vi "Connection Handler Worker.vi"(9 "Additional Data":variant, 10 "connection ID":T1, 11 "TCP Server Refnum":refnum<class "JKI TCP Server.lvclass">) -> ()   [LabVIEW 2020, in "CSM-TCP-Router.lvlib"]
uses:
  CSM-TCP-Router.lvlib
  <vilib>/addons/_JKI.lib/_JKI_lib_TCP_Server.llb/TCP Server Connection Session ID Cluster.ctl
  <vilib>/addons/_JKI.lib/_JKI_lib_TCP_Server.llb/JKI TCP Server.lvclass
  typedef/tcp-msg type.ctl
  20ff867f-262a-4864-b042-c50abd455195.vi
  9f8653f6-ccbf-4dca-88e7-a4c531b7661f.vi
  bd168d05-2ccd-4f69-90c9-be1b4e621865.vi
  316abe05-dd11-44a4-98b3-32ea1594dc48.vi
  a7f8194b-54d4-448d-8a65-d0b66a8fd47c.vi
  8a9da1d4-9237-4126-a3a1-8a9d876b672d.vi
  eb58fbab-51b7-4bfd-aab6-475a21a34b28.vi
  66683ee4-8938-4a2b-95b9-1d8ed72716c9.vi
  <userlib>/_NEVSTOP/Communicable State Machine(CSM)/AdvanceAPI/CSM - Revert Arguments-Safe String.vi
  <userlib>/_NEVSTOP/Communicable State Machine(CSM)/_Support/Common/Trim Single line Text.vi
  <userlib>/_NEVSTOP/Communicable State Machine(CSM)/AdvanceAPI/CSM - Make String Arguments Safe.vi
  <userlib>/_NEVSTOP/Communicable State Machine(CSM)/AdvanceAPI/CSM - Compact Multiple States.vi
  <userlib>/_NEVSTOP/Communicable State Machine(CSM)/addons/API-String-Arugments-Support/_Support/Query Data as API String Arguments(variant).vi
  <userlib>/_NEVSTOP/Communicable State Machine(CSM)/AdvanceAPI/CSM - Keywords.vi
  <userlib>/_NEVSTOP/Communicable State Machine(CSM)/addons/API-String-Arugments-Support/_Support/Data To SingleElementsArray_with_itself_csm.vi
  <userlib>/_NEVSTOP/Communicable State Machine(CSM)/addons/API-String-Arugments-Support/_Support/Data To API String Arguments.vi
  <userlib>/_NEVSTOP/Communicable State Machine(CSM)/addons/API-String-Arugments-Support/_Support/Convert API String Arguments to Data(variant).vi
  <userlib>/_NEVSTOP/Communicable State Machine(CSM)/Communicable State Machine.lvlib
  <userlib>/_NEVSTOP/Communicable State Machine(CSM)/_csmHelper/API with lvcsm Support/CSM-Helper API with lvcsm Support.lvlib
panel:
  out "State History":string
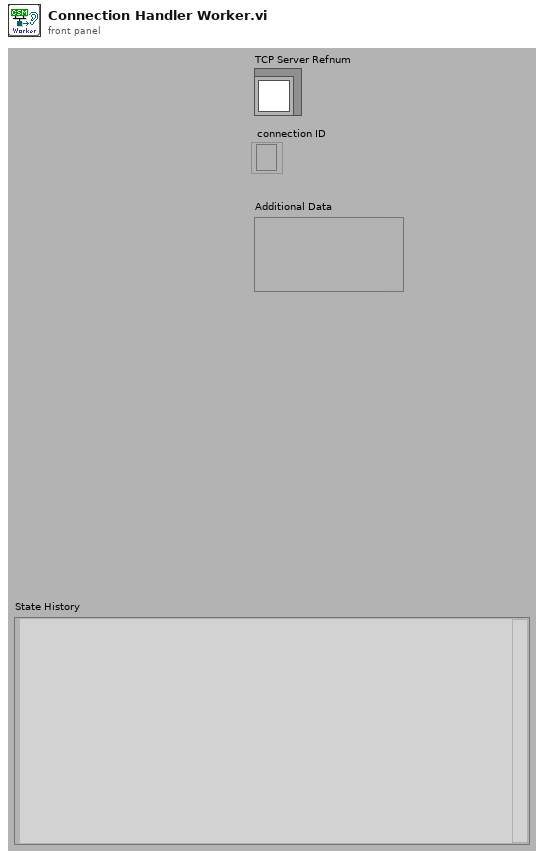
[diagram p1: front panel]
types:
  T1 = typedef "JKI TCP Server.lvclass/TCP Server Connection Session ID Cluster.ctl" = refnum<k5>
  T2 = typedef "CSM-TCP-Router.lvlib/tcp-msg type.ctl" = enum16{"info", "error", "cmd", "resp", "async-resp", "status", "interrupt"}
  T3 = enum32{"Invalid", "Standard", "Closed", "Hidden", "Minimized", "Maximized"}
  T4 = enum32{"invalid app kind", "Development System", "Run Time System", "Student Edition", "Embedded LabVIEW", "Evaluation", "Custom"}
  T5 = typedef "Communicable State Machine.lvlib/_CSM_Response Source Message.ctl" = cluster{"‘State":string, "’Arguments":string, "’Error":errorcluster}
  T6 = cluster{"Current VI Reference":refnum<vi>, "Close Panel on Exit?":bool}
  T7 = cluster{"Core":cluster{"Current VI Reference":refnum<vi>, "Close Panel on Exit?":bool}, "Your Boolean data":bool}
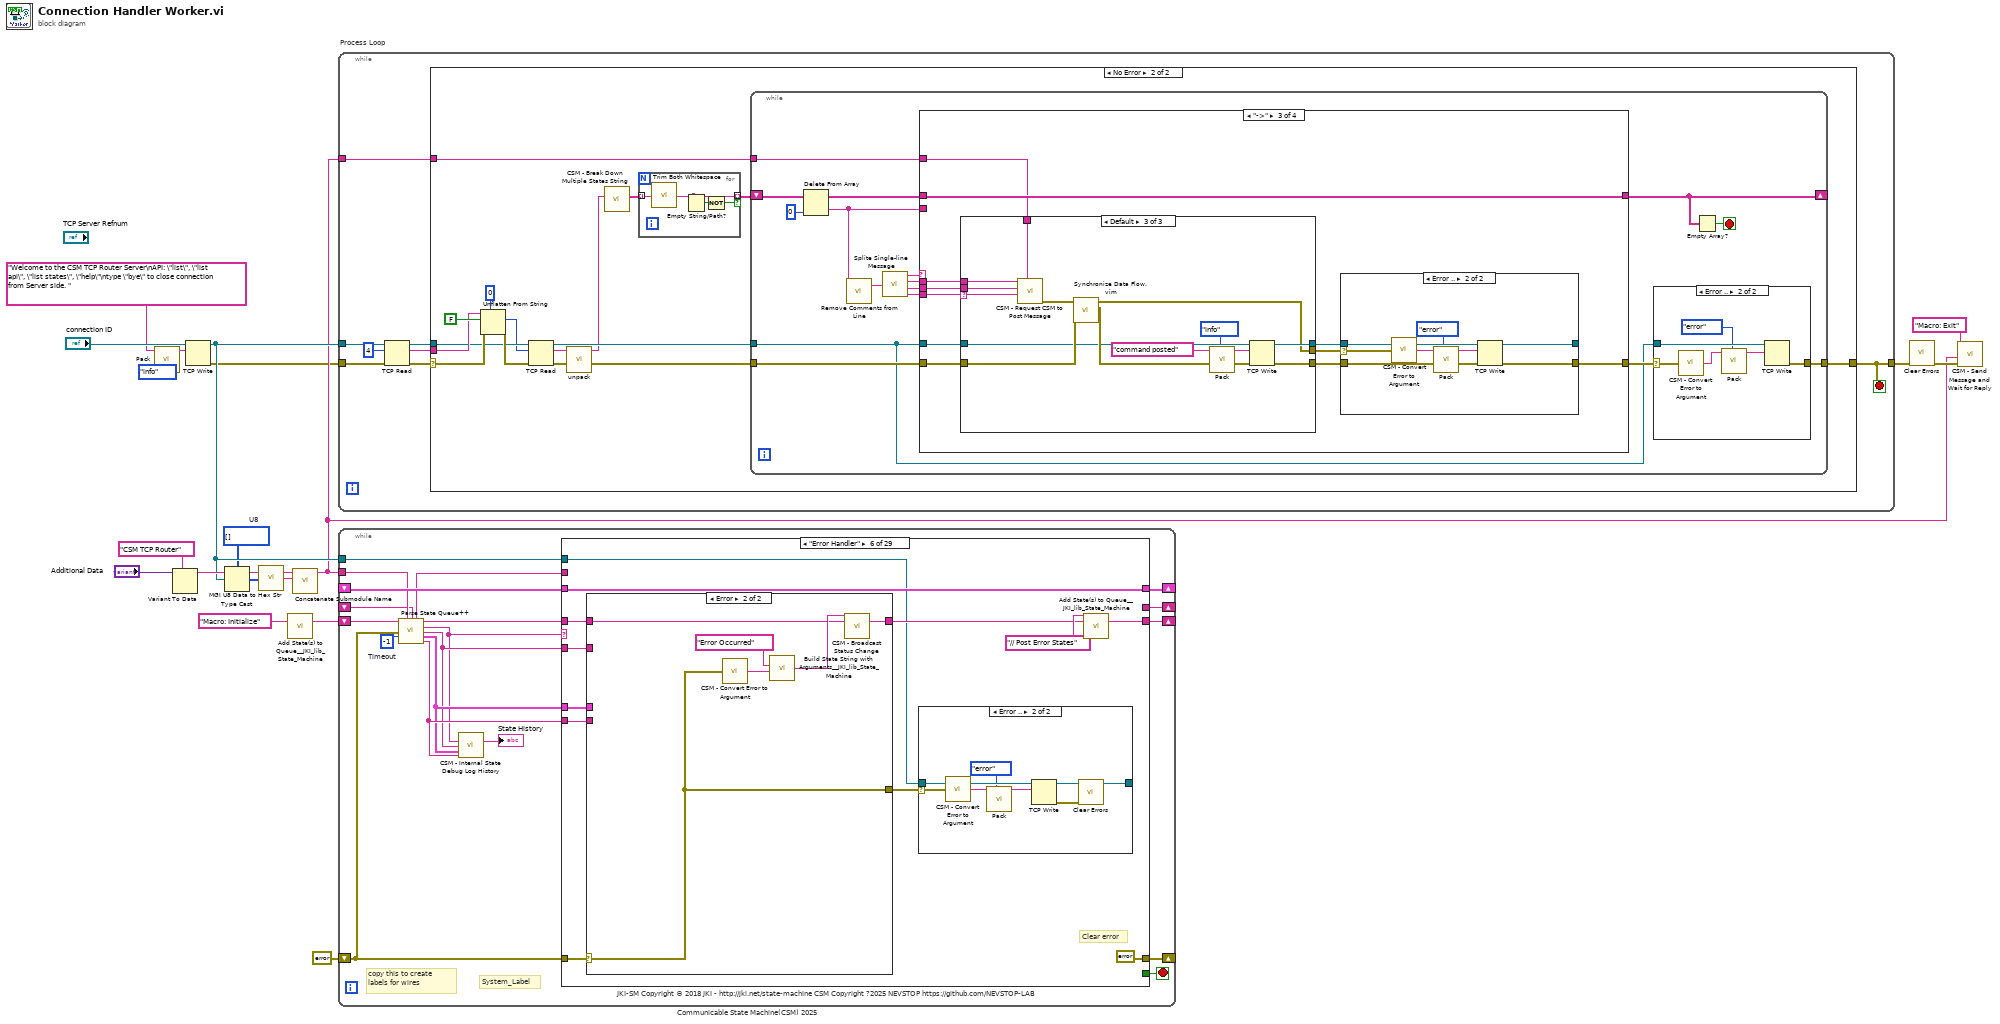
[diagram p0: block diagram]
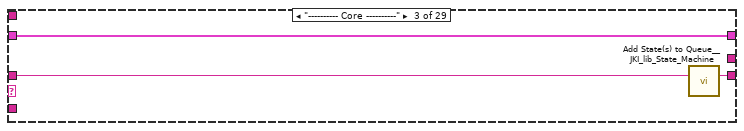
[diagram p4: hidden frame]
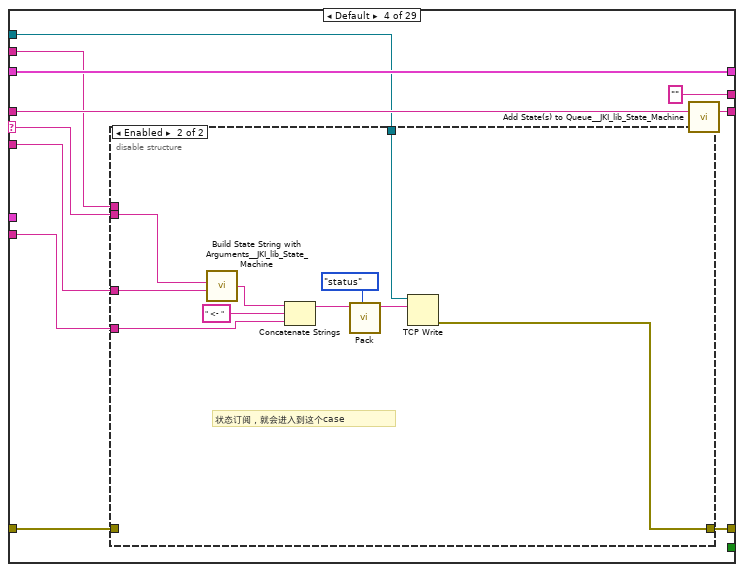
[diagram p5: hidden frame]
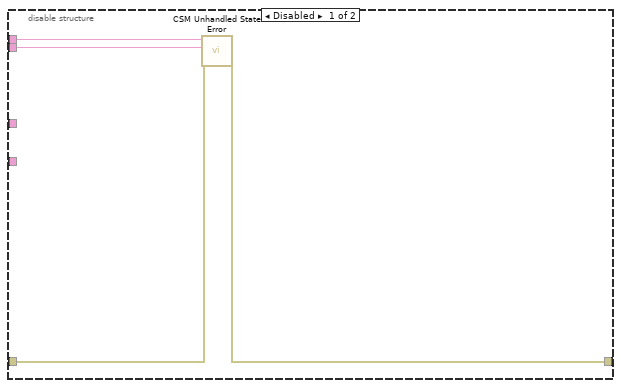
[diagram p6: hidden frame]
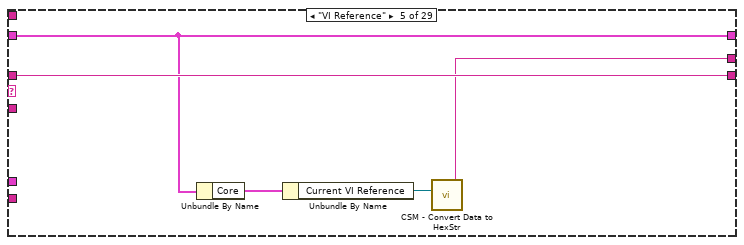
[diagram p7: hidden frame]
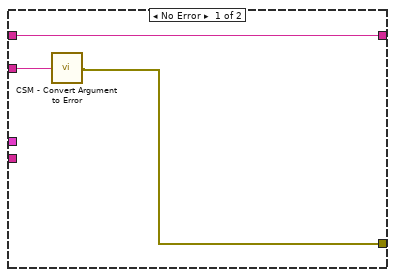
[diagram p9: hidden frame]
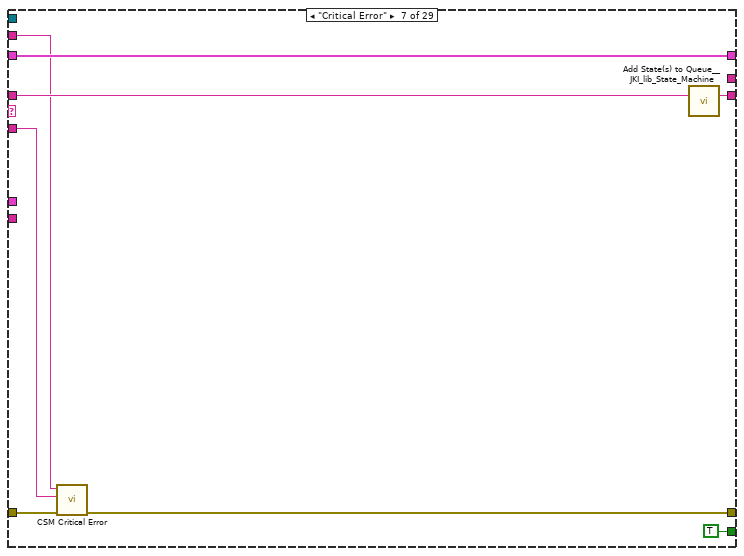
[diagram p10: hidden frame]
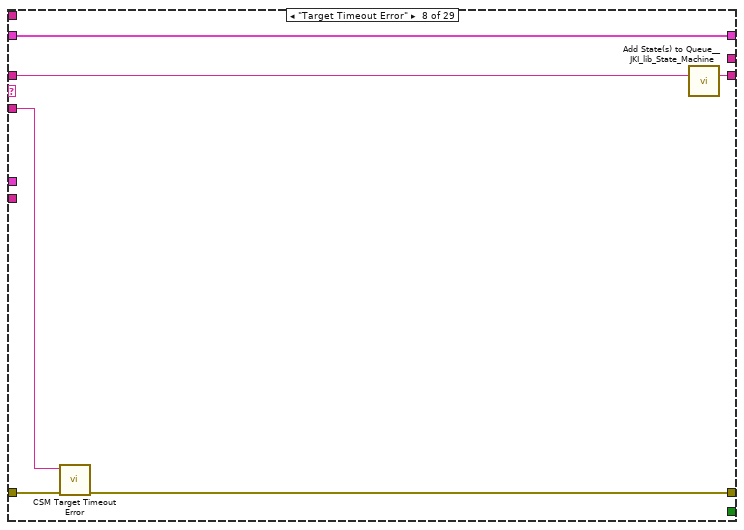
[diagram p11: hidden frame]
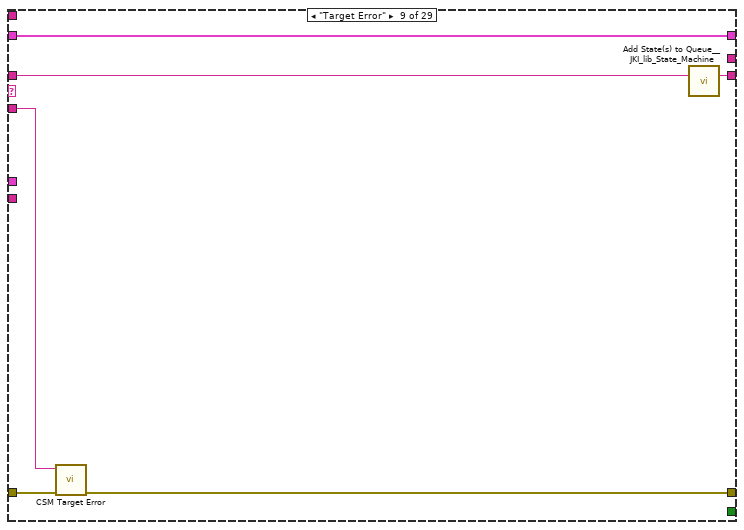
[diagram p12: hidden frame]
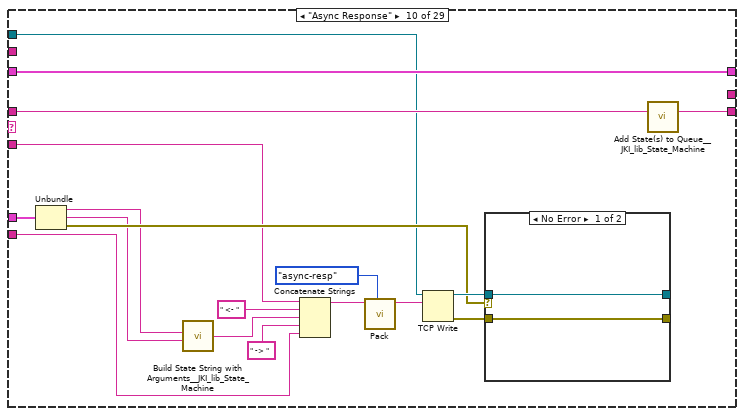
[diagram p13: hidden frame]
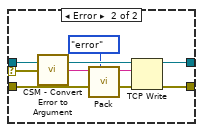
[diagram p14: hidden frame]
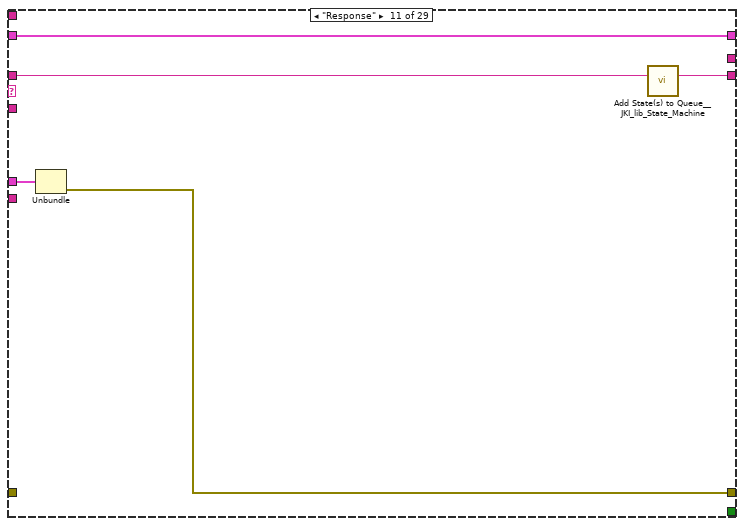
[diagram p15: hidden frame]
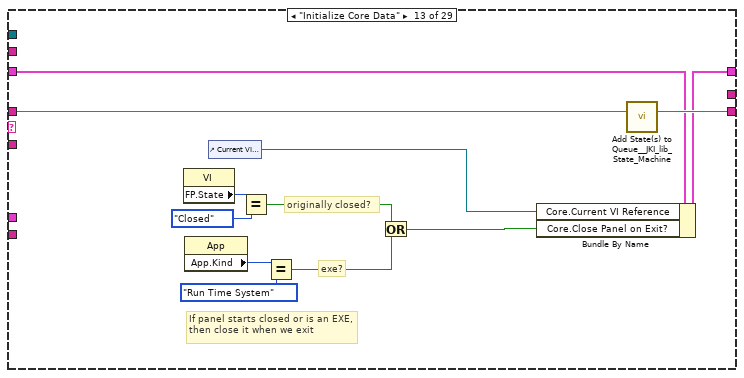
[diagram p17: hidden frame]
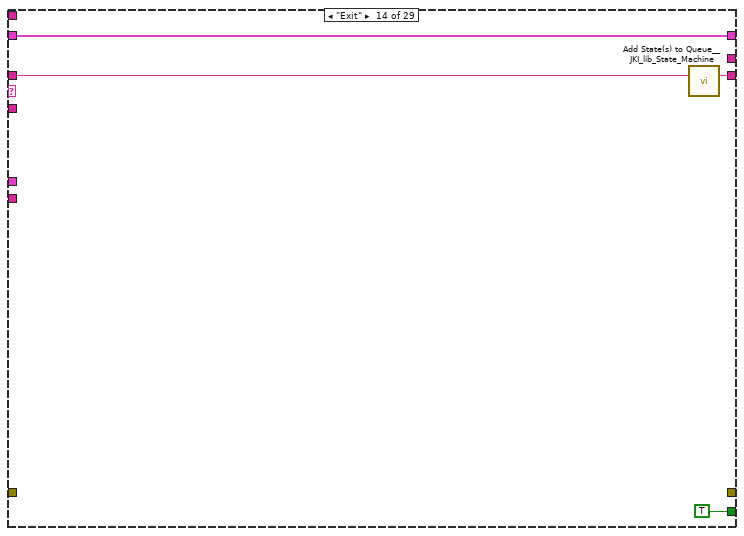
[diagram p18: hidden frame]
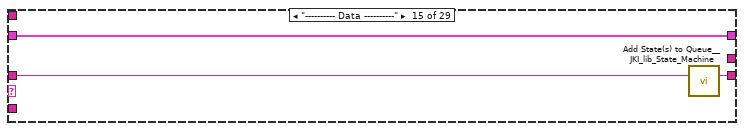
[diagram p19: hidden frame]
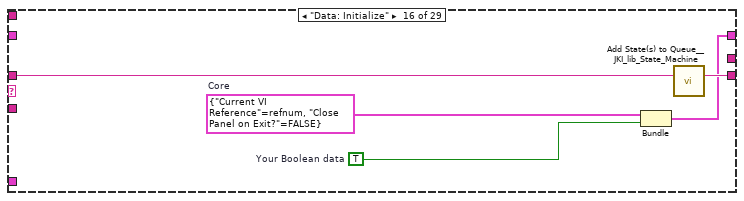
[diagram p20: hidden frame]
diagram:
  w6 = u8[] []  # U8
  n1 = call "Pack.vi"("tcp-message-type"=tcp-msg_type."info", "String"="Welcome to the CSM TCP Router Server\nAPI: \"list\", \"list api\", \"list states\", \"help\"\ntype \"bye\" to close connection from Server side. " ("data in")) -> ("TCP Pack"=w3:string)  [unwired: 9 in]
  n2 = Variant To Data(type="CSM TCP Router" ("Name(\"\" to use uuid)"), Variant="Additional Data") -> (data=w10:string)  [unwired: 1 in, 1 out]
  n3 = TCP Write(connection ID="connection ID", data in=w3) -> (connection ID out=w8:T1, error out=w1:errorcluster)  [unwired: 2 in, 1 out]
  n4 = Type Cast(type=w6, x=w8) -> (*(type *) &x=w5:u8[])
  n5 = call <userlib>:"MGI U8 Data to Hex Str.vi"("u8 Data[]"=w5) -> ("HEX String (0-9,A-F)"=w7:string)
  n6 = call <vilib>:"Add State(s) to Queue__JKI_lib_State_Machine.vi"("State(s) in (\"\")"="Macro: Initialize" ("Init States(\"Macro: Initialize\")")) -> ("States Out"=w16:string)  [unwired: 14 in]
  n7 = call <userlib>:"Concatenate Submodule Name.vi"("name"=w7, "CSM Name"=w10) -> ("submodule name"=w4:string)  [unwired: 9 in]
  n8 = while "Process Loop" {
    tunnel: w8 -> [w27]
    tunnel: [w23] -> w14
    tunnel: w4 -> [w22]
    tunnel: w1 -> [w20]
    stop <- w23 stop-if-true
    n9 = TCP Read(connection ID=w27, bytes to read=4, error in (no error)=w20) -> (connection ID out=w26:T1, data out=w24:string, error out=w25:errorcluster)  [unwired: 2 in]
    n10 = case shown="No Error" w25 {
      selector: w25 -> [w29 w39]
      tunnel: w26 -> [_ w37]
      tunnel: w24 -> [_ w40]
      tunnel: [w28 w46] -> w23
      tunnel: w22 -> [_ w43]
      frame Error {
        n11 = Unbundle By Name(w29) -> ("code"=w30:i32)
        n12 = case shown="56" w30 {
          tunnel: w29 -> [w31 _]
          tunnel: [w31 _] -> w28
          frame 0, Default {
          }
          frame 56 {
          }
        }
      }
      frame No Error {
        n13 = Unflatten From String(type=0, binary string=w40, data includes array or string size? (T)=FALSE, error in (no error)=w39) -> (value=w34:i32, error out=w38:errorcluster)  [unwired: 2 out]
        n14 = TCP Read(connection ID=w37, bytes to read=w34, error in (no error)=w38) -> (connection ID out=w35:T1, data out=w33:string, error out=w36:errorcluster)  [unwired: 2 in]
        n15 = call "unpack.vi"("TCP Pack"=w33) -> ("String"=w32:string)  [unwired: 9 in, 1 out]
        n16 = call <userlib>:"CSM - Break Down Multiple States String.vi"("States"=w32) -> ("Multiple States"=w45:string[])  [unwired: 10 in]
        n17 = for {
          tunnel: w45 -> [w50] mode=indexing
          tunnel: [w49] -> w44 mode=indexing if=w47
          n18 = call <userlib>:"Trim Both Whitespace.vi"("string"=w50) -> ("trimmed string"=w49:string)  [unwired: 1 in]
          n19 = Empty String/Path?(string/path=w49) -> (empty?=w48:bool)
          n20 = Not(x=w48) -> (.not. x?=w47:bool)
        }
        n21 = while {
          tunnel: w35 -> [w53]
          tunnel: w36 -> [w66]
          tunnel: [w54] -> w46
          shift-right: [w56] -> _
          shift-left: w44 -> [w60]
          tunnel: w43 -> [w51]
          stop <- w57 stop-if-true
          n22 = Delete From Array(array=w60, index=0) -> (deleted portion=w52:string, array with subset deleted=w59:string[])  [unwired: 1 in]
          n23 = call <userlib>:"Remove Comments from Line.vi"("single-line text"=w52) -> ("single-line text without comments"=w65:string)  [unwired: 2 in]
          n24 = call <userlib>:"Splite Single-line Message.vi"("single-line text"=w65) -> ("operator"=w64:string, "state"=w63:string, "args"=w62:string, "source/target"=w61:string)  [unwired: 6 in]
          n25 = case shown="\"->\"" w64 {
            selector: w64 -> [w77 _ _ _]
            tunnel: w53 -> [w83 w233 w249 w317]
            tunnel: [w82 w230 w254 w322] -> w55
            tunnel: w66 -> [w81 w226 w252 w320]
            tunnel: w63 -> [w80 w222 w248 w316]
            tunnel: w62 -> [w79 w221 w247 w315]
            tunnel: w61 -> [w78 w223 w246 w314]
            tunnel: [w76 w227 w253 w321] -> w56
            tunnel: w59 -> [w75 w227 w253 w321]
            tunnel: w52 -> [_ _ _ _]
            tunnel: w51 -> [w74 w225 w251 w319]
            frame Default {
              n26 = case shown="\"bye\", \"exit\", \"quit\"" w80 {
                selector: w80 -> [w91 _ _ _ _ _ _]
                tunnel: w83 -> [w94 w101 w113 w121 w147 w173 _]
                tunnel: [w93 errorcluster {"status"=TRUE, "code"=0, "source"=""} ("error out") w108 w120 w146 w172 w205] -> w82
                tunnel: w81 -> [w86 w102 w112 _ _ _ _]
                tunnel: w79 -> [w92 _ _ w116 w142 w168 _]
                tunnel: w78 -> [_ _ _ _ _ _ _]
                tunnel: w77 -> [_ _ _ _ _ _ _]
                tunnel: [w90 w99 w107 w119 w145 w171 w209] -> w76
                tunnel: w75 -> [w90 w99 w107 w119 w145 w171 w209]
                tunnel: w74 -> [_ _ _ w114 w140 w166 w204]
                frame Default {
                  n27 = call <vilib>:"Build State String with Arguments__JKI_lib_State_Machine.vi"("Arguments (\"\")"=w92, "State"=w91) -> ("State with Arguments"=w87:string)  [unwired: 4 in]
                  n28 = Format Into String(format string="You typed \"%s\", which is not recognized as a command", w87) -> (resulting string=w88:string)  [unwired: 2 in, 1 out]
                  n29 = call "Pack.vi"("tcp-message-type"=tcp-msg_type."error", "String"=w88) -> ("TCP Pack"=w85:string)  [unwired: 9 in]
                  n30 = TCP Write(connection ID=w94, data in=w85, error in (no error)=w86) -> (error out=w93:errorcluster)  [unwired: 1 in, 2 out]
                }
                frame "bye", "exit", "quit" {
                  n31 = call "Pack.vi"("tcp-message-type"=tcp-msg_type."info", "String"="Good bye.\r\n" ("data in")) -> ("TCP Pack"=w96:string)  [unwired: 9 in]
                  n32 = TCP Write(connection ID=w101, data in=w96, error in (no error)=w102) -> (connection ID out=w97:T1, error out=w98:errorcluster)  [unwired: 1 in, 1 out]
                  n33 = TCP Close Connection(connection ID=w97, error in (no error)=w98) -> ()  [unwired: 1 in, 2 out]
                }
                frame "list", "list CSM", "List CSMs" {
                  n34 = call <userlib>:"CSM - List Modules.vi"("Error in"=w112) -> ("Error out"=w110:errorcluster, "Module Names"=w111:string[])  [unwired: 9 in]
                  n35 = call "Convert Data To API String Arguments.vim"("error in (no error)"=w110, "data"=w111) -> ("error out"=w109:errorcluster, "String"=w106:string)  [unwired: 6 in]
                  n36 = call "Pack.vi"("tcp-message-type"=tcp-msg_type."resp", "String"=w106) -> ("TCP Pack"=w104:string)  [unwired: 9 in]
                  n37 = TCP Write(connection ID=w113, data in=w104, error in (no error)=w109) -> (error out=w108:errorcluster)  [unwired: 1 in, 2 out]
                }
                frame "list API", "list interface" {
                  n38 = call <userlib>:"CSM - Check If Module Exists.vi"("CSM Name"=w116) -> ("Error out"=w118:errorcluster, "Exist?"=w115:bool, "CSM Name(dup)"=w117:string)  [unwired: 8 in]
                  n39 = case shown="False" w115 {
                    tunnel: w121 -> [w132 w139]
                    tunnel: [w131 w138] -> w120
                    tunnel: w118 -> [w129 _]
                    tunnel: w117 -> [w128 w135]
                    tunnel: w114 -> [w125 _]
                    frame True {
                      n40 = call <userlib>:"Read CSM API with lvcsm Support.vi"("Current Module(\"\" to generate a ID)"=w125, "error in (no error)"=w129, "CSM Name"=w128) -> ("Error out"=w127:errorcluster, "CSMAPI List"=w126:string[])  [unwired: 7 in]
                      n41 = call "Convert Data To API String Arguments.vim"("error in (no error)"=w127, "data"=w126) -> ("error out"=w130:errorcluster, "String"=w123:string)  [unwired: 6 in]
                      n42 = call "Pack.vi"("tcp-message-type"=tcp-msg_type."resp", "String"=w123) -> ("TCP Pack"=w122:string)  [unwired: 9 in]
                      n43 = TCP Write(connection ID=w132, data in=w122, error in (no error)=w130) -> (error out=w131:errorcluster)  [unwired: 1 in, 2 out]
                    }
                    frame False {
                      n44 = Format Into String(format string="\"%s\" module is not existing", w135) -> (resulting string=w136:string)  [unwired: 2 in, 1 out]
                      n45 = call "Pack.vi"("tcp-message-type"=tcp-msg_type."error", "String"=w136) -> ("TCP Pack"=w134:string)  [unwired: 9 in]
                      n46 = TCP Write(connection ID=w139, data in=w134) -> (error out=w138:errorcluster)  [unwired: 2 in, 2 out]
                    }
                  }
                }
                frame "List State", "List States" {
                  n47 = call <userlib>:"CSM - Check If Module Exists.vi"("CSM Name"=w142) -> ("Error out"=w144:errorcluster, "Exist?"=w141:bool, "CSM Name(dup)"=w143:string)  [unwired: 8 in]
                  n48 = case shown="False" w141 {
                    tunnel: w147 -> [w151 w165]
                    tunnel: [w158 w164] -> w146
                    tunnel: w144 -> [w154 _]
                    tunnel: w143 -> [w153 w161]
                    tunnel: w140 -> [w150 _]
                    frame True {
                      n49 = call <userlib>:"Read CSM States with lvcsm Support.vi"("Current Module(\"\" to generate a ID)"=w150, "error in (no error)"=w154, "CSM Name"=w153) -> ("Error out"=w152:errorcluster, "CSMAPI List"=w155:string[])  [unwired: 7 in]
                      n50 = call "Convert Data To API String Arguments.vim"("error in (no error)"=w152, "data"=w155) -> ("error out"=w157:errorcluster, "String"=w156:string)  [unwired: 6 in]
                      n51 = call "Pack.vi"("tcp-message-type"=tcp-msg_type."resp", "String"=w156) -> ("TCP Pack"=w149:string)  [unwired: 9 in]
                      n52 = TCP Write(connection ID=w151, data in=w149, error in (no error)=w157) -> (error out=w158:errorcluster)  [unwired: 1 in, 2 out]
                    }
                    frame False {
                      n53 = Format Into String(format string="\"%s\" module is not existing", w161) -> (resulting string=w162:string)  [unwired: 2 in, 1 out]
                      n54 = call "Pack.vi"("tcp-message-type"=tcp-msg_type."error", "String"=w162) -> ("TCP Pack"=w160:string)  [unwired: 9 in]
                      n55 = TCP Write(connection ID=w165, data in=w160) -> (error out=w164:errorcluster)  [unwired: 2 in, 2 out]
                    }
                  }
                }
                frame "help" {
                  n56 = call <userlib>:"CSM - Check If Module Exists.vi"("CSM Name"=w168) -> ("Error out"=w170:errorcluster, "Exist?"=w167:bool, "CSM Name(dup)"=w169:string)  [unwired: 8 in]
                  n57 = case shown="True" w167 {
                    tunnel: w173 -> [w179 w203]
                    tunnel: [w184 w202] -> w172
                    tunnel: w170 -> [w181 _]
                    tunnel: w169 -> [w180 w199]
                    tunnel: w166 -> [w176 _]
                    frame True {
                      n58 = disable-structure shown="Enabled" {
                        disable-tunnel: w181 -> [w191 w196]
                        disable-tunnel: w180 -> [w190 w195]
                        disable-tunnel: [w188 w193] -> w178
                        disable-tunnel: [w186 w192] -> w177
                        disable-tunnel: w176 -> [w185 w194]
                        frame Disabled {
                          n59 = call <userlib>:"CSM - Module VI Reference.vi"("Current Module(\"\" to generate a ID)"=w185, "error in (no error)"=w191, "CSM Name"=w190) -> ("error out"=w189:errorcluster, "CSM Module VIRef"=w187:refnum<vi>)  [unwired: 7 in]
                          n60 = property class="VI"(reference=w187, error in=w189) -> (error out=w188:errorcluster, "Description"=w186:string)  [unwired: 1 out]
                        }
                        frame Enabled {
                          n61 = call "Read CSM Doc with lvcsm Support.vi"("Current Module(\"\" to generate a ID)"=w194, "error in (no error)"=w196, "CSM Name"=w195) -> ("Error out"=w193:errorcluster, "CSM Doc"=w192:string)  [unwired: 7 in]
                        }
                      }
                      n62 = call "Convert Data To API String Arguments.vim"("error in (no error)"=w178, "data"=w177) -> ("error out"=w183:errorcluster, "String"=w182:string)  [unwired: 6 in]
                      n63 = call "Pack.vi"("tcp-message-type"=tcp-msg_type."resp", "String"=w182) -> ("TCP Pack"=w175:string)  [unwired: 9 in]
                      n64 = TCP Write(connection ID=w179, data in=w175, error in (no error)=w183) -> (error out=w184:errorcluster)  [unwired: 1 in, 2 out]
                    }
                    frame False {
                      n65 = Format Into String(format string="\"%s\" module is not existing", w199) -> (resulting string=w200:string)  [unwired: 2 in, 1 out]
                      n66 = call "Pack.vi"("tcp-message-type"=tcp-msg_type."error", "String"=w200) -> ("TCP Pack"=w198:string)  [unwired: 9 in]
                      n67 = TCP Write(connection ID=w203, data in=w198) -> (error out=w202:errorcluster)  [unwired: 2 in, 2 out]
                    }
                  }
                }
                frame "Refresh lvcsm" {
                  n68 = call <userlib>:"CSM - List Modules.vi"() -> ("Error out"=w208:errorcluster, "Module Names"=w207:string[])  [unwired: 10 in]
                  n69 = for {
                    tunnel: w208 -> [w218]
                    tunnel: w207 -> [w211] mode=indexing
                    tunnel: [w213] -> w206 mode=indexing
                    tunnel: w204 -> [w212]
                    n70 = call <userlib>:"Read CSM States with lvcsm Support.vi"("Current Module(\"\" to generate a ID)"=w212, "error in (no error)"=w218, "Force?(F)"=TRUE, "CSM Name"=w211) -> ("Error out"=w217:errorcluster)  [unwired: 6 in, 1 out]
                    n71 = call <userlib>:"Read CSM API with lvcsm Support.vi"("Current Module(\"\" to generate a ID)"=w212, "error in (no error)"=w217, "Force?(F)"=TRUE, "CSM Name"=w211) -> ("Error out"=w214:errorcluster)  [unwired: 6 in, 1 out]
                    n72 = call "Read CSM Doc with lvcsm Support.vi"("Current Module(\"\" to generate a ID)"=w212, "error in (no error)"=w214, "Force?(F)"=TRUE, "CSM Name"=w211) -> ("Error out"=w213:errorcluster)  [unwired: 6 in, 1 out]
                  }
                  n73 = Merge Errors(w206) -> (w205:errorcluster)
                }
              }
            }
            frame "-@" {
              n74 = call <userlib>:"CSM - Send Message and Wait for Reply.vi"("Current Module(\"\" to generate a ID)"=w225, "Target Module"=w223, "Arguments (\"\")"=w221, "State"=w222) -> ("error out"=w229:errorcluster, "Response"=w224:string)  [unwired: 5 in, 1 out]
              n75 = case shown="\"\"" w224 {
                selector: w224 -> [w234 _]
                tunnel: [w234 ""] -> w228
                frame Default {
                }
                frame "" {
                }
              }
              n76 = call "Pack.vi"("tcp-message-type"=tcp-msg_type."resp", "String"=w228) -> ("TCP Pack"=w220:string)  [unwired: 9 in]
              n77 = TCP Write(connection ID=w233, data in=w220, error in (no error)=w226) -> (connection ID out=w231:T1, error out=w232:errorcluster)  [unwired: 1 in, 1 out]
              n78 = case shown="Error .." w229 {
                selector: w229 -> [_ w242]
                tunnel: w232 -> [w237 w245]
                tunnel: w231 -> [w236 w244]
                tunnel: [w237 w243] -> w230
                tunnel: [w236 w240] -> _
                frame No Error {
                }
                frame Error {
                  n79 = call <userlib>:"CSM - Convert Error to Argument.vi"("error"=w242) -> ("Argument"=w241:string)  [unwired: 4 in]
                  n80 = call "Pack.vi"("tcp-message-type"=tcp-msg_type."error", "String"=w241) -> ("TCP Pack"=w239:string)  [unwired: 9 in]
                  n81 = TCP Write(connection ID=w244, data in=w239, error in (no error)=w245) -> (connection ID out=w240:T1, error out=w243:errorcluster)  [unwired: 1 in, 1 out]
                }
              }
            }
            frame "->" {
              n82 = case shown="Default" w246 {
                selector: w246 -> [_ _ w287]
                tunnel: [w257 w272 w298] -> w256
                tunnel: [w258 w271 w297] -> w255
                tunnel: w252 -> [_ _ w295]
                tunnel: w251 -> [w268 w282 w294]
                tunnel: [_ _ w291] -> w250
                tunnel: w249 -> [w260 w274 w290]
                tunnel: w248 -> [w269 w283 w289]
                tunnel: w247 -> [w270 w284 w288]
                frame "<unregister>" {
                  n83 = call <userlib>:"Parse Unregister Message.vi"("state"=w269, "Module Name"=w268, "args"=w270) -> ("target"=w266:string, "source"=w267:string, "status"=w265:string, "api"=w264:string)  [unwired: 8 in, 1 out]
                  n84 = call <userlib>:"CSM - Unregister Status Change.vi"("CSM Name"=w266, "Source CSM Name (* as Default)"=w267, "Status"=w265, "Response Message (\"*\" as Default)"=w264) -> ("Error out"=w259:errorcluster)  [unwired: 10 in, 1 out]
                  n85 = call "Pack.vi"("tcp-message-type"=tcp-msg_type."info", "String"="done") -> ("TCP Pack"=w262:string)  [unwired: 9 in]
                  n86 = TCP Write(connection ID=w260, data in=w262, error in (no error)=w259) -> (connection ID out=w258:T1, error out=w257:errorcluster)  [unwired: 1 in, 1 out]
                }
                frame "<register>" {
                  n87 = call <userlib>:"Parse Register Message.vi"("state"=w283, "Module Name"=w282, "args"=w284) -> ("target"=w280:string, "source"=w281:string, "status"=w279:string, "api"=w278:string)  [unwired: 8 in, 1 out]
                  n88 = call <userlib>:"CSM - Register Status Change.vi"("CSM Name"=w280, "Source CSM Name (* as Default)"=w281, "Status"=w279, "Response Message (if \"\", same as Source Message)"=w278) -> ("Error out"=w273:errorcluster)  [unwired: 10 in, 1 out]
                  n89 = call "Pack.vi"("tcp-message-type"=tcp-msg_type."info", "String"="done") -> ("TCP Pack"=w276:string)  [unwired: 9 in]
                  n90 = TCP Write(connection ID=w274, data in=w276, error in (no error)=w273) -> (connection ID out=w271:T1, error out=w272:errorcluster)  [unwired: 1 in, 1 out]
                }
                frame Default {
                  n91 = call <userlib>:"CSM - Request CSM to Post Message.vi"("Module Name"=w294, "Target Module(\"\" by Default)"=w287, "Arguments (\"\")"=w288, "State"=w289) -> ("error out"=w292:errorcluster)  [unwired: 7 in]
                  n92 = call "Synchronize Data Flow.vim"("input 2"=w295, "input 1"=w292) -> ("output 2"=w293:errorcluster, "output 1"=w291:errorcluster)  [unwired: 2 in, 2 out]
                  n93 = call "Pack.vi"("tcp-message-type"=tcp-msg_type."info", "String"="command posted") -> ("TCP Pack"=w286:string)  [unwired: 9 in]
                  n94 = TCP Write(connection ID=w290, data in=w286, error in (no error)=w293) -> (connection ID out=w297:T1, error out=w298:errorcluster)  [unwired: 1 in, 1 out]
                }
              }
              n95 = case shown="Error .." w250 {
                selector: w250 -> [_ w305]
                tunnel: w256 -> [w300 w308]
                tunnel: w255 -> [w299 w307]
                tunnel: [w300 w306] -> w254
                tunnel: [w299 w303] -> _
                frame No Error {
                }
                frame Error {
                  n96 = call <userlib>:"CSM - Convert Error to Argument.vi"("error"=w305) -> ("Argument"=w304:string)  [unwired: 4 in]
                  n97 = call "Pack.vi"("tcp-message-type"=tcp-msg_type."error", "String"=w304) -> ("TCP Pack"=w302:string)  [unwired: 9 in]
                  n98 = TCP Write(connection ID=w307, data in=w302, error in (no error)=w308) -> (connection ID out=w303:T1, error out=w306:errorcluster)  [unwired: 1 in, 1 out]
                }
              }
            }
            frame "->|" {
              n99 = call <userlib>:"CSM - Post Message.vi"("Current Module(\"\" to generate a ID)"=w319, "Target Module"=w314, "Arguments (\"\")"=w315, "State"=w316) -> ("error out"=w311:errorcluster)  [unwired: 7 in]
              n100 = call "Synchronize Data Flow.vim"("input 2"=w320, "input 1"=w311) -> ("output 2"=w312:errorcluster, "output 1"=w318:errorcluster)  [unwired: 2 in, 2 out]
              n101 = call "Pack.vi"("tcp-message-type"=tcp-msg_type."info", "String"="<Command Posted>") -> ("TCP Pack"=w310:string)  [unwired: 9 in]
              n102 = TCP Write(connection ID=w317, data in=w310, error in (no error)=w312) -> (connection ID out=w323:T1, error out=w324:errorcluster)  [unwired: 1 in, 1 out]
              n103 = case shown="Error .." w318 {
                selector: w318 -> [_ w331]
                tunnel: w324 -> [w326 w334]
                tunnel: w323 -> [w325 w333]
                tunnel: [w326 w332] -> w322
                tunnel: [w325 w329] -> _
                frame No Error {
                }
                frame Error {
                  n104 = call <userlib>:"CSM - Convert Error to Argument.vi"("error"=w331) -> ("Argument"=w330:string)  [unwired: 4 in]
                  n105 = call "Pack.vi"("tcp-message-type"=tcp-msg_type."error", "String"=w330) -> ("TCP Pack"=w328:string)  [unwired: 9 in]
                  n106 = TCP Write(connection ID=w333, data in=w328, error in (no error)=w334) -> (connection ID out=w329:T1, error out=w332:errorcluster)  [unwired: 1 in, 1 out]
                }
              }
            }
          }
          n107 = case shown="Error .." w55 {
            selector: w55 -> [w67 w70]
            tunnel: w53 -> [_ w73]
            tunnel: [w67 w72] -> w54
            frame No Error {
            }
            frame Error {
              n108 = call <userlib>:"CSM - Convert Error to Argument.vi"("error"=w70) -> ("Argument"=w71:string)  [unwired: 4 in]
              n109 = call "Pack.vi"("tcp-message-type"=tcp-msg_type."error", "String"=w71) -> ("TCP Pack"=w69:string)  [unwired: 9 in]
              n110 = TCP Write(connection ID=w73, data in=w69) -> (error out=w72:errorcluster)  [unwired: 2 in, 2 out]
            }
          }
          n111 = Empty Array?(array=w56) -> (empty?=w57:bool)
        }
      }
    }
  }
  n112 = while "Communicable State Machine(CSM) 2025" {
    shift-right: [w348] -> _
    shift-left: _ -> [w347]
    shift-right: [w351] -> _
    shift-left: errorcluster {"status"=FALSE, "code"=0, "source"=""} ("error out") -> [w337]
    shift-right: [w350] -> _
    shift-left: w16 -> [w352]
    tunnel: w4 -> [w344]
    shift-right: [w345] -> _
    shift-left: _ -> [w339]
    tunnel: w8 -> [w335]
    stop <- w349 stop-if-true
    w346 = -1  # Timeout
    # "copy this to create labels for wires"
    # "System_Label"
    # "JKI-SM Copyright © 2018 JKI - http://jki.net/state-machine CSM Copyright ?2025 NEVSTOP https://github.com/NEVSTOP-LAB"
    n113 = call <userlib>:"Parse State Queue++.vi"("State Queue"=w352, "Name(\"\" to use uuid)"=w344, "Response Arguments"=w339, "Previous Error"=w337, "Dequeue Timeout(0ms)"=w346) -> ("Name Used"=w338:string, "Remaining States"=w353:string, "Current State"=w340:string, "Arguments"=w341:string, ">> Response Source Message >>"=w342:T5, ">> Source CSM >>"=w343:string)  [unwired: 5 in]
    n114 = call <userlib>:"CSM - Internal State Debug Log History.vi"("State"=w340, "Arguments (\"\")"=w341, ">> Response Source Message >>"=w342, "Source (\"\")"=w343) -> ("Debug Log"=→"State History":string)  [unwired: 11 in]
    n115 = case shown="\"Error Handler\"" w340 {
      selector: w340 -> [_ _ _ w366 _ _ _ _ _ _ _ _ _ _ _ _ _ _ _ _ _ _ _ _ _ _ _ _ _]
      tunnel: w353 -> [w354 w357 w360 w369 w390 w396 w426 w432 w438 w455 w470 w474 w486 w490 w493 w498 w504 w509 w511 w516 w519 w523 w527 w529 w532 w536 w541 w545 w548]
      tunnel: w341 -> [_ _ _ w362 _ w395 w420 w429 w435 w447 _ _ _ _ _ _ w499 w508 _ _ _ _ _ _ _ w534 _ _ _]
      tunnel: w347 -> [w355 w356 w358 w367 w387 w401 w424 w430 w436 w456 w471 w473 w480 w488 w491 _ w503 w507 w510 w512 w517 w521 w525 w528 w531 w535 w539 w543 w546]
      tunnel: [_ _ _ w371 _ errorcluster {"status"=FALSE, "code"=0, "source"=""} ("error out") w427 w428 w434 _ w468 _ _ _ _ _ w500 w505 _ w513 _ _ _ _ _ _ _ _ _] -> w351
      tunnel: w337 -> [_ _ _ w370 _ w399 w422 w433 w439 _ _ _ _ _ _ _ _ _ _ _ _ _ _ _ _ _ _ _ _]
      tunnel: [w354 w357 w359 w368 w390 w397 w425 w431 w437 w457 w472 w474 w485 w489 w492 w497 w504 w509 w511 w515 w518 w522 w526 w529 w532 w536 w540 w544 w547] -> w350
      tunnel: [_ _ _ _ _ _ TRUE _ _ _ _ _ _ TRUE _ _ _ _ _ _ _ _ _ _ _ _ _ _ _] -> w349
      tunnel: [w355 w356 w358 w367 w387 w401 w424 w430 w436 w456 w471 w473 w484 w488 w491 w496 w502 w506 w510 w512 w517 w521 w525 w528 w531 w535 w539 w543 w546] -> w348
      tunnel: w343 -> [_ _ _ w361 _ w394 _ _ _ w440 _ _ _ _ _ _ _ _ _ _ _ _ _ _ _ _ _ _ _]
      tunnel: w342 -> [_ _ _ _ _ w393 _ _ _ w454 w469 _ _ _ _ _ _ _ _ _ _ _ _ _ _ _ _ _ _]
      tunnel: [_ _ _ "" w386 _ _ _ _ _ _ _ _ _ _ _ w501 _ _ _ _ _ _ _ "API1 Response" w533 _ "Action Finished" _] -> w345
      tunnel: w338 -> [_ _ _ w364 _ _ w421 _ _ _ _ _ _ _ _ _ _ _ _ _ _ _ _ _ _ _ _ _ _]
      tunnel: w335 -> [_ _ _ w363 _ w391 _ _ _ w448 _ _ _ _ _ _ _ _ _ _ _ _ _ _ _ _ _ _ _]
      frame "", "Idle" {
      }
      frame "CSM Documentation" {
      }
      frame "---------- Core ----------" {
        n116 = call <vilib>:"Add State(s) to Queue__JKI_lib_State_Machine.vi"("State(s) in (\"\")"=w360) -> ("States Out"=w359:string)  [unwired: 14 in]
      }
      frame Default {
        n117 = disable-structure shown="Enabled" {
          disable-tunnel: [w375 w376] -> w371
          disable-tunnel: w370 -> [w374 _]
          disable-tunnel: w366 -> [w373 w380]
          disable-tunnel: w364 -> [w372 _]
          disable-tunnel: w363 -> [_ w381]
          disable-tunnel: w362 -> [_ w379]
          disable-tunnel: w361 -> [_ w377]
          frame Disabled {
            n118 = call <userlib>:"CSM Unhandled State Error.vi"("error in (no error)"=w374, "Current State"=w373, "CSM Name"=w372) -> ("error out"=w375:errorcluster)  [unwired: 8 in]
          }
          frame Enabled {
            # "状态订阅，就会进入到这个case"
            n119 = call <vilib>:"Build State String with Arguments__JKI_lib_State_Machine.vi"("Arguments (\"\")"=w379, "State"=w380) -> ("State with Arguments"=w378:string)  [unwired: 4 in]
            n120 = Concatenate Strings(w378, " <- " ("string"), w377) -> (w383:string)
            n121 = call "Pack.vi"("tcp-message-type"=tcp-msg_type."status", "String"=w383) -> ("TCP Pack"=w385:string)  [unwired: 9 in]
            n122 = TCP Write(connection ID=w381, data in=w385) -> (error out=w376:errorcluster)  [unwired: 2 in, 2 out]
          }
        }
        n123 = call <vilib>:"Add State(s) to Queue__JKI_lib_State_Machine.vi"("State(s) in (\"\")"=w369) -> ("States Out"=w368:string)  [unwired: 14 in]
      }
      frame "VI Reference" {
        n124 = Unbundle By Name(w387) -> ("Core"=w389:T6)
        n125 = Unbundle By Name(w389) -> ("Current VI Reference"=w388:refnum<vi>)
        n126 = call <userlib>:"CSM - Convert Data to HexStr.vi"("Variant"=w388) -> ("HEX String (0-9,A-F)"=w386:string)  [unwired: 8 in]
      }
      frame "Error Handler" {
        # "Clear error"
        n127 = case shown="Error" w399 {
          selector: w399 -> [_ w414]
          tunnel: [w413 w416] -> w398
          tunnel: w396 -> [w413 w415]
          tunnel: w395 -> [w412 _]
          tunnel: w394 -> [_ _]
          tunnel: w393 -> [_ _]
          tunnel: [w411 w414] -> w392
          frame No Error {
            n128 = call <userlib>:"CSM - Convert Argument to Error.vi"("Argument"=w412) -> ("error"=w411:errorcluster)  [unwired: 4 in]
          }
          frame Error {
            n129 = call <userlib>:"CSM - Convert Error to Argument.vi"("error"=w414) -> ("Argument"=w418:string)  [unwired: 4 in]
            n130 = call <vilib>:"Build State String with Arguments__JKI_lib_State_Machine.vi"("Arguments (\"\")"=w418, "State"="Error Occurred" ("Status with Arguments")) -> ("State with Arguments"=w417:string)  [unwired: 4 in]
            n131 = call <userlib>:"CSM - Broadcast Status Change.vi"("Status with Arguments"=w417, "State Queue"=w415) -> ("Remaining States"=w416:string)  [unwired: 13 in]
          }
        }
        n132 = case shown="Error .." w392 {
          selector: w392 -> [_ w408]
          tunnel: w391 -> [w403 w410]
          tunnel: [w403 w406] -> _
          frame No Error {
          }
          frame Error {
            n133 = call <userlib>:"CSM - Convert Error to Argument.vi"("error"=w408) -> ("Argument"=w407:string)  [unwired: 4 in]
            n134 = call "Pack.vi"("tcp-message-type"=tcp-msg_type."error", "String"=w407) -> ("TCP Pack"=w405:string)  [unwired: 9 in]
            n135 = TCP Write(connection ID=w410, data in=w405) -> (connection ID out=w406:T1, error out=w409:errorcluster)  [unwired: 2 in, 1 out]
            n136 = call <vilib>:"Clear Errors.vi"("error in (no error)"=w409) -> ()  [unwired: 5 in, 2 out]
          }
        }
        n137 = call <vilib>:"Add State(s) to Queue__JKI_lib_State_Machine.vi"("State(s) in Front (\"\")"="// Post Error States", "State(s) in (\"\")"=w398) -> ("States Out"=w397:string)  [unwired: 13 in]
      }
      frame "Critical Error" {
        n138 = call <userlib>:"CSM Critical Error.vi"("error in (no error)"=w422, "Arugments(as Reason)"=w420, "CSM Name"=w421) -> ("error out"=w427:errorcluster)  [unwired: 8 in]
        n139 = call <vilib>:"Add State(s) to Queue__JKI_lib_State_Machine.vi"("State(s) in (\"\")"=w426) -> ("States Out"=w425:string)  [unwired: 14 in]
      }
      frame "Target Timeout Error" {
        n140 = call <userlib>:"CSM Target Timeout Error.vi"("error in (no error)"=w433, "Arguments(as CSM Name)"=w429) -> ("error out"=w428:errorcluster)  [unwired: 9 in]
        n141 = call <vilib>:"Add State(s) to Queue__JKI_lib_State_Machine.vi"("State(s) in (\"\")"=w432) -> ("States Out"=w431:string)  [unwired: 14 in]
      }
      frame "Target Error" {
        n142 = call <userlib>:"CSM Target Error.vi"("error in (no error)"=w439, "Arguments(as CSM Name)"=w435) -> ("error out"=w434:errorcluster)  [unwired: 9 in]
        n143 = call <vilib>:"Add State(s) to Queue__JKI_lib_State_Machine.vi"("State(s) in (\"\")"=w438) -> ("States Out"=w437:string)  [unwired: 14 in]
      }
      frame "Async Response" {
        n144 = Unbundle(w454) -> ("‘State"=w444:string, "’Arguments"=w443:string, "’Error"=w449:errorcluster)
        n145 = call <vilib>:"Build State String with Arguments__JKI_lib_State_Machine.vi"("Arguments (\"\")"=w443, "State"=w444) -> ("State with Arguments"=w442:string)  [unwired: 4 in]
        n146 = Concatenate Strings(w447, " <- " ("string"), w442, " -> " ("string"), w440) -> (w446:string)
        n147 = call "Pack.vi"("tcp-message-type"=tcp-msg_type."async-resp", "String"=w446) -> ("TCP Pack"=w453:string)  [unwired: 9 in]
        n148 = TCP Write(connection ID=w448, data in=w453) -> (connection ID out=w452:T1, error out=w451:errorcluster)  [unwired: 2 in, 1 out]
        n149 = case shown="No Error" w449 {
          selector: w449 -> [_ w464]
          tunnel: w451 -> [w459 w467]
          tunnel: w452 -> [w458 w466]
          tunnel: [w459 w465] -> _
          tunnel: [w458 w462] -> _
          frame No Error {
          }
          frame Error {
            n150 = call <userlib>:"CSM - Convert Error to Argument.vi"("error"=w464) -> ("Argument"=w463:string)  [unwired: 4 in]
            n151 = call "Pack.vi"("tcp-message-type"=tcp-msg_type."error", "String"=w463) -> ("TCP Pack"=w461:string)  [unwired: 9 in]
            n152 = TCP Write(connection ID=w466, data in=w461, error in (no error)=w467) -> (connection ID out=w462:T1, error out=w465:errorcluster)  [unwired: 1 in, 1 out]
          }
        }
        n153 = call <vilib>:"Add State(s) to Queue__JKI_lib_State_Machine.vi"("State(s) in (\"\")"=w455) -> ("States Out"=w457:string)  [unwired: 14 in]
      }
      frame "Response" {
        n154 = Unbundle(w469) -> ("’Error"=w468:errorcluster)  [unwired: 2 out]
        n155 = call <vilib>:"Add State(s) to Queue__JKI_lib_State_Machine.vi"("State(s) in (\"\")"=w470) -> ("States Out"=w472:string)  [unwired: 14 in]
      }
      frame "Async Message Posted" {
      }
      frame "Initialize Core Data" {
        # "originally closed?"
        # "exe?"
        # "If panel starts closed or is an EXE, then close it when we exit"
        n156 = property class="VI"() -> ("FP.State"=w477:T3)  [unwired: 2 in, 2 out]
        n157 = property class="App"() -> ("App.Kind"=w483:T4)  [unwired: 2 in, 2 out]
        n158 = control-ref of="Current VI Reference"() -> (w478:refnum<vi>)
        n159 = Equal?(x=w477, y=T3."Closed" ("Front Panel Window:State")) -> (x = y?=w475:bool)
        n160 = Equal?(x=w483, y=T4."Run Time System" ("Application:Kind")) -> (x = y?=w481:bool)
        n161 = Or(x=w475, y=w481) -> (x .or. y?=w479:bool)
        n162 = Bundle By Name(cluster=w480, "Core.Current VI Reference"=w478, "Core.Close Panel on Exit?"=w479) -> (w484:T7)
        n163 = call <vilib>:"Add State(s) to Queue__JKI_lib_State_Machine.vi"("State(s) in (\"\")"=w486) -> ("States Out"=w485:string)  [unwired: 14 in]
      }
      frame "Exit" {
        n164 = call <vilib>:"Add State(s) to Queue__JKI_lib_State_Machine.vi"("State(s) in (\"\")"=w490) -> ("States Out"=w489:string)  [unwired: 14 in]
      }
      frame "---------- Data ----------" {
        n165 = call <vilib>:"Add State(s) to Queue__JKI_lib_State_Machine.vi"("State(s) in (\"\")"=w493) -> ("States Out"=w492:string)  [unwired: 14 in]
      }
      frame "Data: Initialize" {
        w494 = T6 {"Current VI Reference"=refnum, "Close Panel on Exit?"=FALSE}  # Core
        w495 = TRUE  # Your Boolean data
        n166 = Bundle("Core"=w494, "Your Boolean data"=w495) -> (w496:T7)  [unwired: 1 in]
        n167 = call <vilib>:"Add State(s) to Queue__JKI_lib_State_Machine.vi"("State(s) in (\"\")"=w498) -> ("States Out"=w497:string)  [unwired: 14 in]
      }
      frame "Data: Get Configuration", "Data: Get Internal Data" {
        n168 = call "Query Data as API String Arguments.vim"("Setting Name"=w499, "Internal Data"=w503) -> ("error"=w500:errorcluster, "Setting as String"=w501:string, "Internal Data(dup)"=w502:T7)  [unwired: 7 in]
      }
      frame "Data: Set Configuration" {
        n169 = call "Convert API String Arguments to Data.vim"("Type"=w507, "String"=w508) -> ("error"=w505:errorcluster, "Data"=w506:T7)  [unwired: 6 in]
      }
      frame "Data: Update Indicators" {
      }
      frame "Data: Cleanup" {
        n170 = Unbundle By Name(w512) -> ("Core.Current VI Reference"=w514:refnum<vi>)
        n171 = Close Reference(reference=w514) -> (error out=w513:errorcluster)  [unwired: 1 in]
        n172 = call <vilib>:"Add State(s) to Queue__JKI_lib_State_Machine.vi"("State(s) in (\"\")"=w516) -> ("States Out"=w515:string)  [unwired: 14 in]
      }
      frame "---------- Macro ----------" {
        n173 = call <vilib>:"Add State(s) to Queue__JKI_lib_State_Machine.vi"("State(s) in (\"\")"=w519) -> ("States Out"=w518:string)  [unwired: 14 in]
      }
      frame "Macro: Initialize" {
        n174 = call <vilib>:"Add State(s) to Queue__JKI_lib_State_Machine.vi"("State(s) in Front (\"\")"="Data: Initialize\nInitialize Core Data\nData: Update Indicators", "State(s) in (\"\")"=w523) -> ("States Out"=w522:string)  [unwired: 13 in]
      }
      frame "Macro: Exit" {
        n175 = call <vilib>:"Add State(s) to Queue__JKI_lib_State_Machine.vi"("State(s) in Front (\"\")"="Data: Cleanup\nExit", "State(s) in (\"\")"=w527) -> ("States Out"=w526:string)  [unwired: 13 in]
      }
      frame "---------- API ----------" {
      }
      frame "API: API1" {
      }
      frame "API: API2" {
        # "unpack Hex String  to Variant\nif complex parameter is needed."
        n176 = call <userlib>:"CSM - Convert HexStr to Data.vi"("HEX String"=w534) -> ()  [unwired: 7 in, 2 out]
        n177 = disable-structure shown="Enabled" {
          disable-tunnel: [w537 "API2 Response"] -> w533
          frame Disabled {
            # "pack variant to hexstr \nif complex response is needed."
            # "complex Response"
            n178 = call <userlib>:"CSM - Convert Data to HexStr.vi"() -> ("HEX String (0-9,A-F)"=w537:string)  [unwired: 9 in]
          }
          frame Enabled {
          }
        }
      }
      frame "---------- Action ----------" {
        n179 = call <vilib>:"Add State(s) to Queue__JKI_lib_State_Machine.vi"("State(s) in (\"\")"=w541) -> ("States Out"=w540:string)  [unwired: 14 in]
      }
      frame "Action: Send Sync Message" {
        n180 = call <vilib>:"Add State(s) to Queue__JKI_lib_State_Machine.vi"("State(s) in (\"\")"=w545) -> ("States Out"=w544:string)  [unwired: 14 in]
      }
      frame "Action: Action2" {
        n181 = call <vilib>:"Add State(s) to Queue__JKI_lib_State_Machine.vi"("State(s) in (\"\")"=w548) -> ("States Out"=w547:string)  [unwired: 14 in]
      }
    }
  }
  n182 = call <vilib>:"Clear Errors.vi"("error in (no error)"=w14) -> ("error out"=w13:errorcluster)  [unwired: 5 in, 1 out]
  n183 = call <userlib>:"CSM - Send Message and Wait for Reply.vi"("Error In (no error)"=w13, "Target Module"=w4, "State"="Macro: Exit") -> ()  [unwired: 6 in, 3 out]
